vi "Get Plugin Components.vi"(8 "error in (no error)":errorcluster, 11 "Item Ref in":T1 format="%.0x") -> (0 "error out":errorcluster, 1 "all found?":bool, 2 "Plugin Components":refnum<class "Component.lvclass">[](array[class]), 3 "Item Ref out":T1 format="%.0x")   [LabVIEW 2019, in "DSF System Explorer.lvlib"]
uses:
  DSF System Explorer.lvlib
  Shared/DSF Shared.lvlib
  <vilib>/NI VeriStand/Custom Device API/Custom Device Item Ref.ctl
  <vilib>/NI VeriStand/Custom Device API/Custom Device API.lvlib
  DSF Core.lvlibp/Classes/Component/Component.lvclass
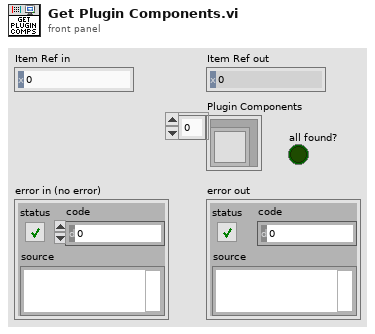
[diagram p1: front panel]
types:
  T1 = typedef "Custom Device API.lvlib/Custom Device Item Ref.ctl" = u64
  T2 = typedef "DSF Core.lvlibp/Plugin Configuration.lvclass/Core Plugin Configuration.ctl" = cluster{"name":string, "components":string[], "cycle timing":T3}
  T3 = typedef "DSF Core.lvlibp/DSF Timing Info.ctl" = cluster{"priority":u64, "decimation":u64, "offset":u64}
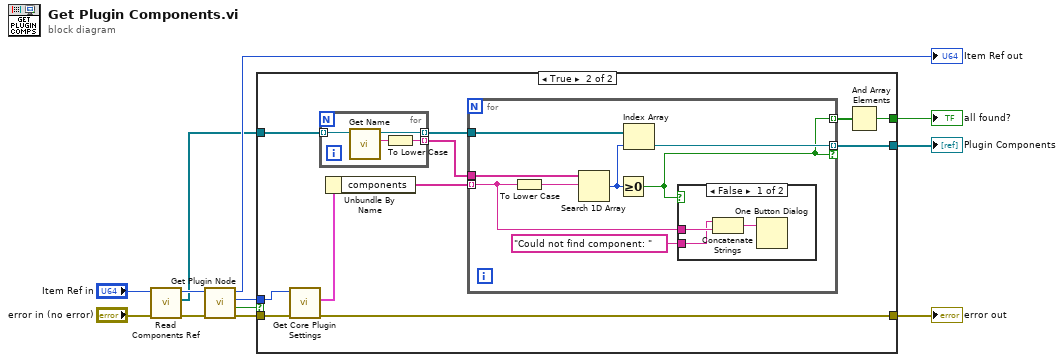
[diagram p0: block diagram]
diagram:
  n1 = call "Read Components Ref.vi"("error in (no error)"="error in (no error)", "Item Ref in"="Item Ref in") -> ("error out"=w7:errorcluster, "Components"=w4:refnum<class "Component.lvclass">[], "Item Ref out"=w6:T1)  [unwired: 7 in]
  n2 = call "Get Plugin Node.vi"("error in (no error)"=w7, "Item Ref in"=w6) -> ("error out"=w12:errorcluster, "found?"=w11:bool, "Plugin Ref"=w10:T1, "Item Ref out"=→"Item Ref out":T1)  [unwired: 6 in]
  n3 = case shown="True" w11 {
    tunnel: w12 -> [w13 w24]
    tunnel: w10 -> [_ w23]
    tunnel: w4 -> [_ w18]
    tunnel: [_ w20] -> w3
    tunnel: [w13 w19] -> w2
    tunnel: [_ w14] -> w1
    frame False {
    }
    frame True {
      n4 = call "Get Core Plugin Settings.vi"("error in (no error)"=w24, "Item Ref in"=w23) -> ("error out"=w19:errorcluster, "plugin configuration"=w22:T2)  [unwired: 7 in, 1 out]
      n5 = for {
        tunnel: w18 -> [w28] mode=indexing
        tunnel: [w25] -> w17 mode=indexing
        tunnel: [w26] -> w16 mode=indexing
        n6 = call "Get Name.vi"("Component in"=w28) -> ("name"=w27:string, "Component out"=w26:refnum<class "Component.lvclass">)  [unwired: 9 in]
        n7 = To Lower Case(string=w27) -> (all lower case string=w25:string)
      }
      n8 = Unbundle By Name(w22) -> ("components"=w21:string[])
      n9 = for {
        tunnel: w21 -> [w31] mode=indexing
        tunnel: [w30] -> w20 mode=indexing if=w29
        tunnel: w17 -> [w35]
        tunnel: w16 -> [w34]
        tunnel: [w29] -> w15 mode=indexing
        n10 = To Lower Case(string=w31) -> (all lower case string=w32:string)
        n11 = Search 1D Array(1D array=w35, element=w32) -> (index of element=w33:i32)  [unwired: 1 in]
        n12 = Greater Or Equal To 0?(x=w33) -> (x >= 0?=w29:bool)
        n13 = Index Array(array=w34, index=w33) -> (element=w30:refnum<class "Component.lvclass">)
        n14 = case shown="False" w29 {
          tunnel: w31 -> [w39 _]
          tunnel: "Could not find component: " -> [w38 _]
          frame False {
            n15 = Concatenate Strings(w38, w39) -> (w37:string)
            n16 = One Button Dialog(message=w37) -> ()  [unwired: 1 in, 1 out]
          }
          frame True {
          }
        }
      }
      n17 = And Array Elements(Boolean array=w15) -> (logical AND=w14:bool)
    }
  }
  "error out" <- w2
  "Plugin Components" <- w3
  "all found?" <- w1
